vi "IAmGLF-NotARefnum.vi"(11 "View in":refnum<class "View.lvclass">) -> (2 "Not A Valid Refnum?":bool=TRUE, 3 "View out":refnum<class "View.lvclass">)   [LabVIEW 2024, in "GLF.lvlib" / "View.lvclass"]
doc: "<B>Summary</B>\nReturns <B>True</B> if the class is invalid."
uses:
  View.lvclass
  View.lvclass/View.ctl
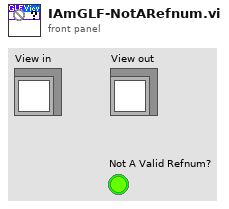
[diagram p1: front panel]
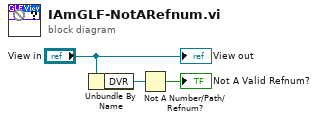
[diagram p0: block diagram]
diagram:
  n1 = Unbundle By Name("View in") -> ("DVR"=w2:refnum<data-value>)
  n2 = Not A Number/Path/Refnum?(number/path/refnum=w2) -> (NaN/Path/Refnum?=→"Not A Valid Refnum?":bool)
  "View out" <- "View in"
